vi "J1939 Claim With ECU.vi"(8 "error in (no error)":errorcluster, 10 "SAE J1939:ECU":refnum<k21>, 11 "XNET Session":refnum<k21>) -> (0 "error out":errorcluster, 2 "Assigned J1939 Address":u8, 3 "XNET Session Out":refnum<k21>)   [LabVIEW 2014, in "J1939 runtime.lvclass"]
uses:
  J1939 runtime.lvclass
  <resource>/objmgr/xnet.rc
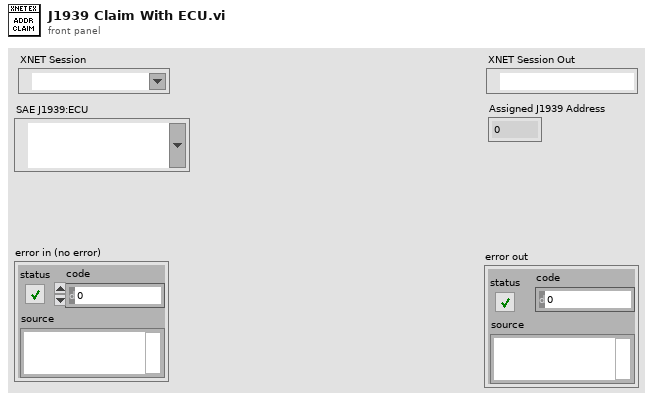
[diagram p1: front panel]
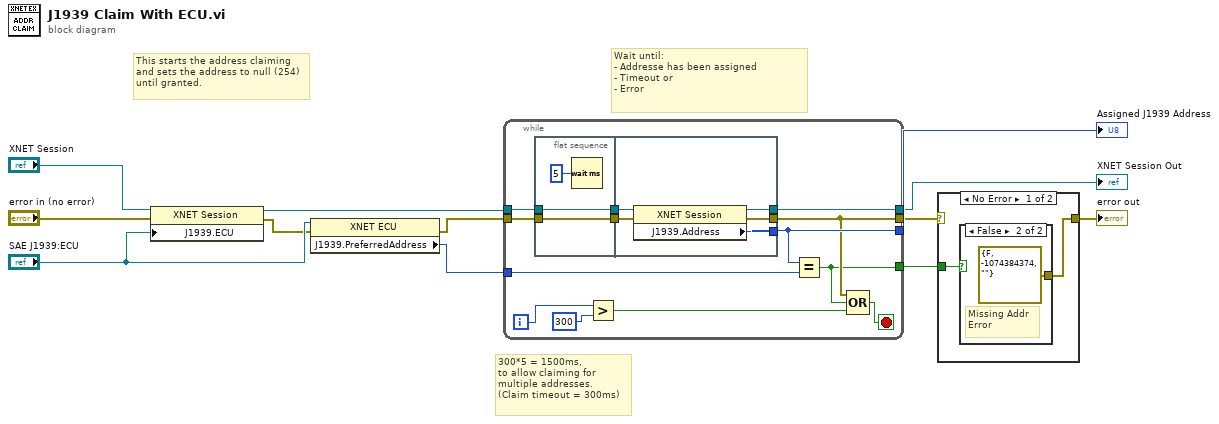
[diagram p0: block diagram]
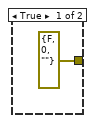
[diagram p2: hidden frame]
diagram:
  # "This starts the address claiming\nand sets the address to null (254)\nuntil granted."
  # "300*5 = 1500ms,\nto allow claiming for \nmultiple addresses.\n(Claim timeout = 300ms)"
  # "Wait until:\n- Addresse has been assigned\n- Timeout or\n- Error"
  n1 = property class="XNET Session"(reference="XNET Session", error in="error in (no error)", "J1939.ECU"="SAE J1939:ECU") -> (reference out=w5:refnum<k21>, error out=w3:errorcluster)
  n2 = property class="XNET ECU"(reference="SAE J1939:ECU", error in=w3) -> (error out=w2:errorcluster, "J1939.PreferredAddress"=w1:u32)  [unwired: 1 out]
  n3 = while {
    tunnel: [w23] -> w12
    tunnel: w2 -> [w25]
    tunnel: [w17] -> w9
    tunnel: w5 -> [w22]
    tunnel: [w20] -> w11
    tunnel: w1 -> [w14]
    tunnel: [w13] -> w10
    i -> [w19]
    stop <- w16 stop-if-true
    n4 = flat-sequence {
      tunnel: w25 -> [w28]
      tunnel: [w28] -> w24
      tunnel: w22 -> [w26]
      tunnel: [w26] -> w21
      tunnel: [w33] -> w23
      tunnel: w24 -> [w32]
      tunnel: [w31] -> w17
      tunnel: w21 -> [w30]
      tunnel: [w29] -> w20
      frame #0 {
        n5 = Wait (ms)(milliseconds to wait=u32 5) -> ()  [unwired: 1 out]
      }
      frame #1 {
        n6 = property class="XNET Session"(reference=w30, error in=w32) -> (reference out=w29:refnum<k21>, error out=w31:errorcluster, "J1939.Address"=w33:u8)
      }
    }
    n7 = Greater?(x=w19, y=300) -> (0:w15:bool)
    n8 = Equal?(x=w23, y=w14) -> (x = y?=w13:bool)
    n9 = Compound Arithmetic op=OR(w17, w13, w15) -> (w16:bool)
  }
  "Assigned J1939 Address" <- w12
  "XNET Session Out" <- w11
  n10 = case shown="No Error" w9 {
    selector: w9 -> [_ w38]
    tunnel: w10 -> [w35 _]
    tunnel: [w34 w38] -> w8
    frame No Error {
      n11 = case shown="False" w35 {
        tunnel: [errorcluster {"status"=FALSE, "code"=0, "source"=""} ("error out") errorcluster {"status"=FALSE, "code"=-1074384374, "source"=""} ("error out")] -> w34
        frame True {
        }
        frame False {
          # "Missing Addr\nError"
        }
      }
    }
    frame Error {
    }
  }
  "error out" <- w8
